vi "OAT Demodulate Multiple Orders (Multi Channels).vi"(0 "Y":dbl[][](array[numeric]) format="%.2f", 2 "reset? (True)":bool=TRUE, 3 "zero delay? (F)":bool, 5 "samples/rev":dbl=2.0 format="%.2f", 7 "samples/rev wanted":dbl=1.0 format="%.2f", 9 "orders (1.0)":dbl[](array[numeric])=[1.0] format="%.2f", 11 "time stamps in":dbl[](array[numeric]) format="%.2f", 12 "phase setting":T3, 13 "order info":T1 {"stop band attenuation" items=["72 dB", "96 dB", "120 dB"]; "bandwidth [order]" format="%.2f"}) -> (4 "magnitudes (RMS)":dbl[][][](array[numeric]) format="%.2f", 6 "phase lag":dbl[][][](array[numeric]) format="%.2f", 10 "samples/rev":dbl format="%.2f", 14 "speed profile":T2 {"speed [RPM]" format="%.2f"; "time [s]" format="%.2f"}, 15 "error out":errorcluster)   [LabVIEW 2017, in "SoundVib_Resampling.lvlib"]
uses:
  <vilib>/addons/Sound and Vibration/Order Analysis/Resample Order Tracking/SoundVib_Resampling.lvlib
  <vilib>/addons/Sound and Vibration/Order Analysis/Tach Process/SubVIs/speed profile.ctl
  <vilib>/addons/Sound and Vibration/Order Analysis/Tach Process/SoundVib_TachProcess.lvlib
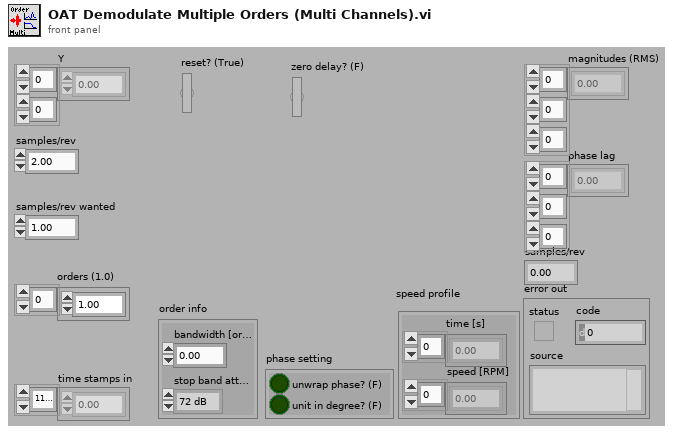
[diagram p1: front panel]
types:
  T1 = cluster{"bandwidth [order]":dbl, "stop band attenuation":u16}
  T2 = typedef "SoundVib_TachProcess.lvlib/speed profile.ctl" = cluster{"time [s]":dbl[], "speed [RPM]":dbl[]}
  T3 = cluster{"unwrap phase? (F)":bool, "unit in degree? (F)":bool}
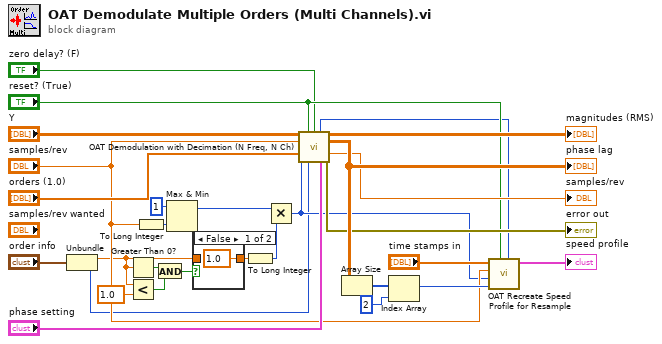
[diagram p0: block diagram]
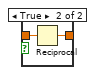
[diagram p2: hidden frame]
diagram:
  n1 = Unbundle("order info") -> ("bandwidth [order]"=w4:dbl, "stop band attenuation"=w3:u16)
  n2 = Greater Than 0?(x=w4) -> (x > 0?=w12:bool)
  n3 = Less?(x=w4, y=1.0) -> (x < y?=w11:bool)
  n4 = To Long Integer(number="samples/rev") -> (32bit integer=w25:i32)
  n5 = And(x=w12, y=w11) -> (x .and. y?=w10:bool)
  n6 = Max & Min(x=1, y=w25) -> (max(x,y)=w7:i32)  [unwired: 1 out]
  n7 = case shown="False" w10 {
    tunnel: w4 -> [_ w32]
    tunnel: [1.0 w31] -> w9
    frame False {
    }
    frame True {
      n8 = Reciprocal(x=w32) -> (1/x=w31:dbl)
    }
  }
  n9 = To Long Integer(number=w9) -> (32bit integer=w8:i32)
  n10 = Multiply(x=w7, y=w8) -> (x*y=w6:i32)
  n11 = call <vilib>:"OAT Demodulation with Decimation (N Freq, N Ch).vi"("x[n]"="Y", "reset? (True)"="reset? (True)", "zero delay? (F)"="zero delay? (F)", "fs"="samples/rev", "fc [Hz]"="orders (1.0)", "decimation factor"=w6, "stop band attenuation"=w3, "phase setting"="phase setting") -> ("lags"=w2:i32, "magnitudes (RMS)"=→"magnitudes (RMS)":dbl[][][], "phase lag"=w23:dbl[][][], "new fs [Hz]"=→"samples/rev":dbl, "error out"=→"error out":errorcluster)  [unwired: 3 in]
  "phase lag" <- w23
  n12 = Array Size(array=w23) -> (size(s)=w22:i32[])
  n13 = Index Array(array=w22, index=2) -> (element=w18:i32)
  n14 = call <vilib>:"OAT Recreate Speed Profile for Resample.vi"("lags"=w2, "init/continue (init:T)"="reset? (True)", "output length"=w18, "decimation factor"=w6, "sample / rev"="samples/rev", "time stamps in"="time stamps in") -> ("speed profile"=→"speed profile":T2)  [unwired: 5 in]
